vi "Wave2D_Check Input_BC.vi"(8 "error in (no error)":errorcluster, 10 "Domain":T2={"t"={"initial t"=0.0, "final t"=1.0, "# of t-points"=11}, "x"={"start x"=0.0, "end x"=1.0, "# of x-points"=11}, "y"={"start y"=0.0, "end y"=1.0, "# of y-points"=11}}, 11 "Boundary Condition":cluster{"type":T1, "Value":dbl[][]}[](array[cluster]) {"type" items=["Dirichlet", "Neumann"]}) -> (0 "error out":errorcluster)   [LabVIEW 2017, in "NI_PDE.lvlib"]
uses:
  <vilib>/gmath/NI_PDE.lvlib
  <vilib>/gmath/pde.llb/Common/PDE_BC Type.ctl
  <vilib>/gmath/pde.llb/Common/PDE_Error.ctl
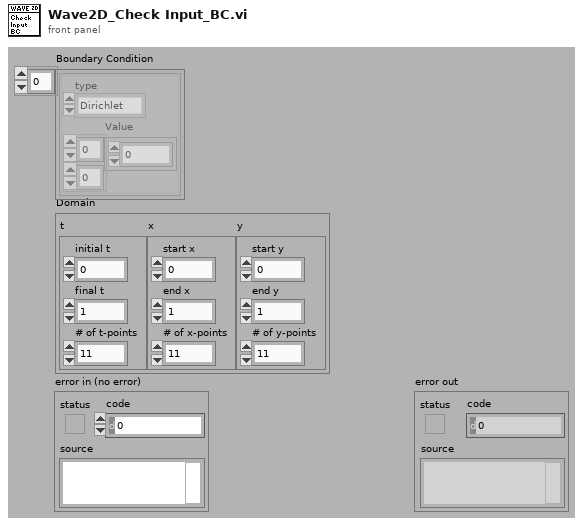
[diagram p1: front panel]
types:
  T1 = typedef "NI_PDE.lvlib/PDE_BC Type.ctl" = i32
  T2 = cluster{"t":cluster{"initial t":dbl, "final t":dbl, "# of t-points":i32}, "x":cluster{"start x":dbl, "end x":dbl, "# of x-points":i32}, "y":cluster{"start y":dbl, "end y":dbl, "# of y-points":i32}}
  T3 = typedef "NI_PDE.lvlib/PDE_Error.ctl" = enum16{"No Error", "k is zero", "End point <= start point", "# of time steps < 2", "# of spatial points < 3", "# of grid < 1 for FEM", "# of boundary < 3 for FEM", "Incompatible RHS size", "Incompatible BC size", "Incompatible IC size", "PDE class conflict", "RHS class conflict", "Domain class conflict", "BC class conflict", "IC class conflict"}
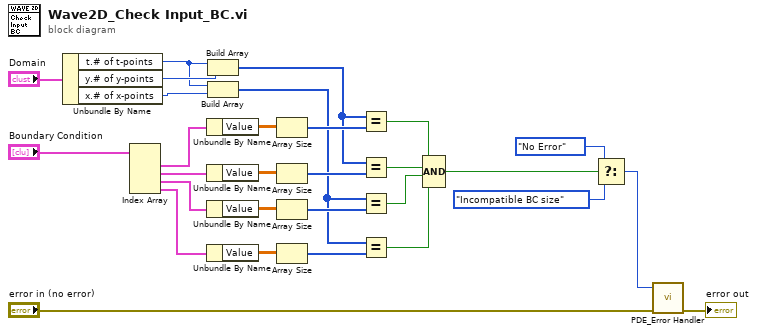
[diagram p0: block diagram]
diagram:
  n1 = Unbundle By Name("Domain") -> ("t.# of t-points"=w21:i32, "y.# of y-points"=w22:i32, "x.# of x-points"=w20:i32)
  n2 = Index Array(array="Boundary Condition") -> (element #1=w23:cluster{"type":T1, "Value":dbl[][]}, element #2=w18:cluster{"type":T1, "Value":dbl[][]}, element #3=w13:cluster{"type":T1, "Value":dbl[][]}, element #4=w10:cluster{"type":T1, "Value":dbl[][]})  [unwired: 4 in]
  n3 = Unbundle By Name(w23) -> ("Value"=w26:dbl[][])
  n4 = Unbundle By Name(w18) -> ("Value"=w19:dbl[][])
  n5 = Unbundle By Name(w13) -> ("Value"=w14:dbl[][])
  n6 = Unbundle By Name(w10) -> ("Value"=w12:dbl[][])
  n7 = Build Array(w21, w22) -> (w16:i32[])
  n8 = Build Array(w21, w20) -> (w9:i32[])
  n9 = Array Size(array=w26) -> (size(s)=w25:i32[])
  n10 = Array Size(array=w19) -> (size(s)=w17:i32[])
  n11 = Array Size(array=w14) -> (size(s)=w15:i32[])
  n12 = Array Size(array=w12) -> (size(s)=w11:i32[])
  n13 = Equal?(x=w16, y=w25) -> (x = y?=w7:bool)
  n14 = Equal?(x=w16, y=w17) -> (x = y?=w8:bool)
  n15 = Equal?(x=w9, y=w15) -> (x = y?=w6:bool)
  n16 = Equal?(x=w9, y=w11) -> (x = y?=w5:bool)
  n17 = Compound Arithmetic op=AND(w7, w8, w6, w5) -> (w4:bool)
  n18 = Select(t=PDE_Error."No Error" ("PDE error"), s=w4, f=PDE_Error."Incompatible BC size" ("PDE error")) -> (s? t:f=w2:T3)
  n19 = call <vilib>:"PDE_Error Handler.vi"("error in (no error)"="error in (no error)", "PDE error"=w2) -> ("error out"=→"error out":errorcluster)  [unwired: 9 out]
